vi "KE237_CommandsGlobal.vi"() -> ()   [LabVIEW 2018, in "KE237.lvclass"]
uses:
  KE237.lvclass
panel:
  in  "Keithley 237 GPIB Setup":T1={"Instrument name"="Keithley 237", "Command \"Reset\""="J0X", "Command \"Initialise\""="K0Y0G5,1,0N0R1O0T4,0,0,0F0,0P3S3B0,0,0L%1.6f,%dX", "Command \"Arm\""="B0,0,0N1X", "Command \"SetVolts\""="B%3.2f,0,0F0,0H0X", "Command \"Compliance?\""="", "Command \"Standby\""="B0,0,0N0X", "Command \"Read Current\""=""}
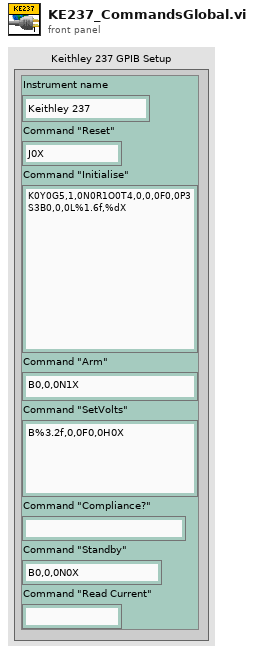
[diagram p1: front panel]
types:
  T1 = cluster{"Instrument name":string, "Command \"Reset\"":string, "Command \"Initialise\"":string, "Command \"Arm\"":string, "Command \"SetVolts\"":string, "Command \"Compliance?\"":string, "Command \"Standby\"":string, "Command \"Read Current\"":string}
diagram:
